vi "Gui_Read_INI.vi"(0 "Key":string, 3 "error in (no error)":errorcluster, 4 "Section":string) -> (7 "value":string caption="valeur", 10 "error out":errorcluster caption="sortie d'erreur")   [LabVIEW 2017]
uses:
  <vilib>/Utility/config.llb/Read Key (String).vi
  <vilib>/Utility/config.llb/NI_LVConfig.lvlib
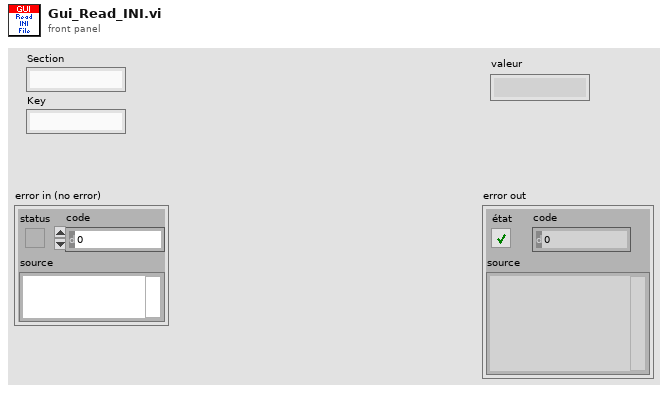
[diagram p1: front panel]
types:
  T1 = typedef "NI_LVConfig.lvlib/Config Data RefNum.ctl" = refnum<k1>
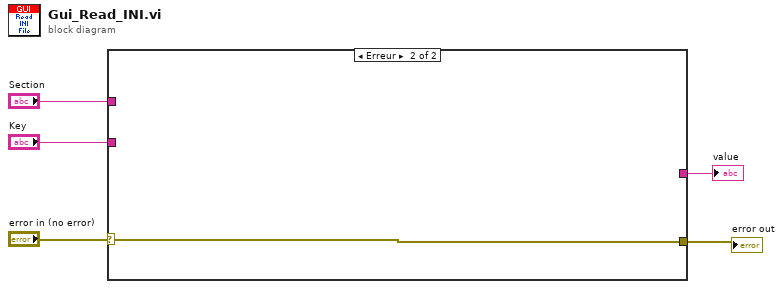
[diagram p0: block diagram]
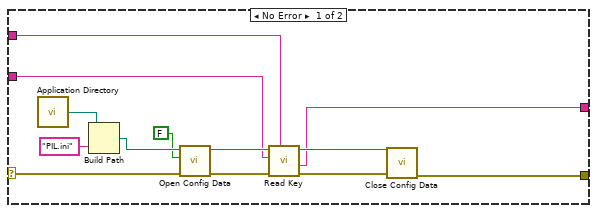
[diagram p2: hidden frame]
diagram:
  n1 = case shown="Erreur" "error in (no error)" {
    selector: "error in (no error)" -> [w18 w19]
    tunnel: [w15 w19] -> w5
    tunnel: "Key" -> [w9 _]
    tunnel: "Section" -> [w8 _]
    tunnel: [w6 _] -> w1
    frame No Error {
      n2 = call <vilib>:"Application Directory.vi"() -> ("Application Directory"=w14:path)
      n3 = Build Path(base path=w14, name or relative path="PIL.ini" ("nom ou chemin relatif")) -> (appended path=w12:path)
      n4 = call <vilib>:"Open Config Data.vi"("error in (no error)"=w18, "create file if necessary (T)"=FALSE, "configuration file path"=w12) -> ("error out"=w17:errorcluster, "refnum"=w10:T1)  [unwired: 6 in, 1 out]
      n5 = call-poly <vilib>:"Read Key.vi"("section"=w8, "error in (no error)"=w17, "key"=w9, "refnum"=w10) -> ("error out"=w16:errorcluster, "value"=w6:string, "refnum out"=w7:T1)  [unwired: 4 in, 1 out]
      n6 = call <vilib>:"Close Config Data.vi"("error in (no error)"=w16, "refnum"=w7) -> ("error out"=w15:errorcluster)  [unwired: 8 in, 1 out]
    }
    frame Error {
    }
  }
  "error out" <- w5
  "value" <- w1
